vi "Preprocess_Data_for_TDMS.vi"(9 "Super Loop Index":i32, 10 "Previous Cluster":T2={"Meas Pressure"=[], "Meas Flowrate"=[], "Current Time"=0.0, "Start Time"=0.0, "Ref Pressure"=[], "Ref Flowrate"=[], "Flowrate Limits"={"Max"=300.0, "Min"=0.0}, "Chan 1 Gains"={"Kp"=0.0, "Ti"=0.0, "Td"=0.0}, "Chan 2 Gains"={"Kp"=0.0, "Ti"=0.0, "Td"=0.0}, "Chan 3 Gains"={"Kp"=0.0, "Ti"=0.0, "Td"=0.0}}, 11 "Current Cluster":T2={"Meas Pressure"=[], "Meas Flowrate"=[], "Current Time"=0.0, "Start Time"=0.0, "Ref Pressure"=[], "Ref Flowrate"=[], "Flowrate Limits"={"Max"=300.0, "Min"=0.0}, "Chan 1 Gains"={"Kp"=0.0, "Ti"=0.0, "Td"=0.0}, "Chan 2 Gains"={"Kp"=0.0, "Ti"=0.0, "Td"=0.0}, "Chan 3 Gains"={"Kp"=0.0, "Ti"=0.0, "Td"=0.0}}) -> (1 "appended array":bool[](array[boolean]), 2 "Contoler Change?":bool, 3 "output cluster":T1)   [LabVIEW 2021]
panel:
  out "initialized array":dbl[][](array[numeric])
  out "P":dbl[][](array[numeric])
  out "P array":dbl[][](array[numeric])
  out "Meas Pressure":dbl[](array[numeric])
  out "Ref Pressure":dbl[](array[numeric])
  out "FR":dbl[][](array[numeric])
  out "Ref P":dbl[][](array[numeric])
  out "Ref FR":dbl[][](array[numeric])
  out "Control":dbl[][](array[numeric])
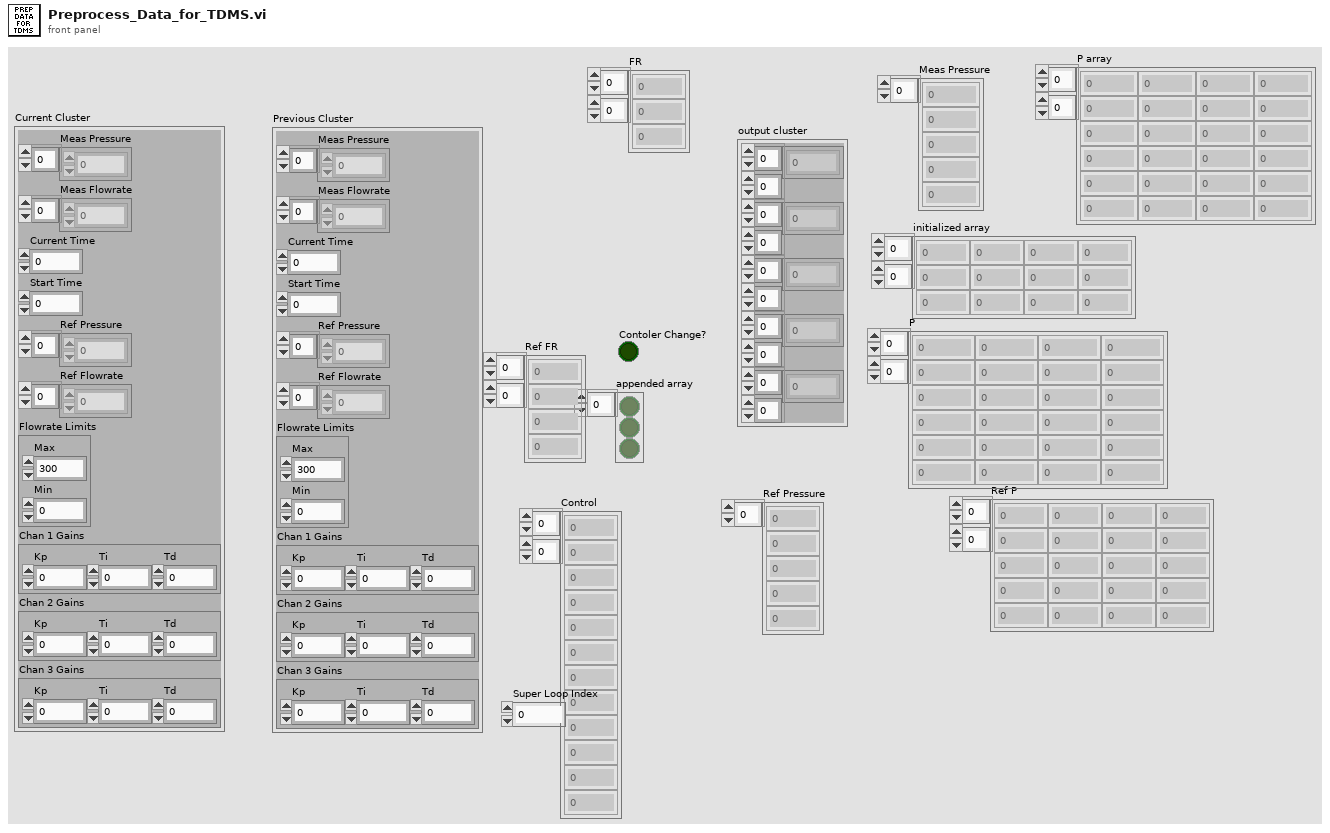
[diagram p1: front panel]
types:
  T1 = cluster{dbl[][], dbl[][], dbl[][], dbl[][], dbl[][]}
  T2 = cluster{"Meas Pressure":dbl[], "Meas Flowrate":dbl[], "Current Time":dbl, "Start Time":dbl, "Ref Pressure":dbl[], "Ref Flowrate":dbl[], "Flowrate Limits":cluster{"Max":dbl, "Min":dbl}, "Chan 1 Gains":cluster{"Kp":dbl, "Ti":dbl, "Td":dbl}, "Chan 2 Gains":cluster{"Kp":dbl, "Ti":dbl, "Td":dbl}, "Chan 3 Gains":cluster{"Kp":dbl, "Ti":dbl, "Td":dbl}}
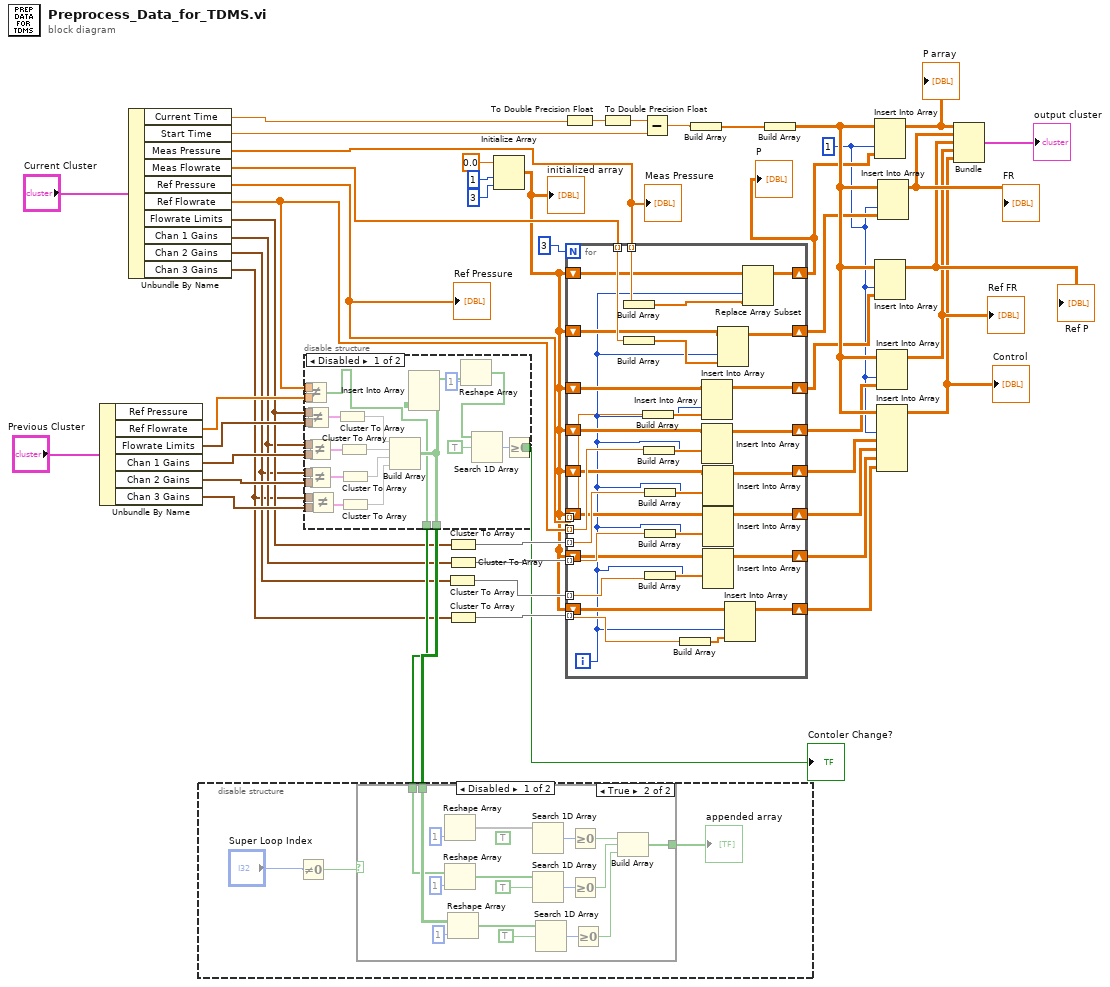
[diagram p0: block diagram]
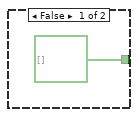
[diagram p3: hidden frame]
diagram:
  w1 = 1 ("disabled index (col)")
  n1 = Unbundle By Name("Previous Cluster") -> ("Ref Flowrate"=w37:dbl[], "Flowrate Limits"=w32:cluster{"Max":dbl, "Min":dbl}, "Chan 1 Gains"=w31:cluster{"Kp":dbl, "Ti":dbl, "Td":dbl}, "Chan 2 Gains"=w30:cluster{"Kp":dbl, "Ti":dbl, "Td":dbl}, "Chan 3 Gains"=w29:cluster{"Kp":dbl, "Ti":dbl, "Td":dbl})  [unwired: 1 out]
  n2 = Unbundle By Name("Current Cluster") -> ("Current Time"=w40:dbl, "Start Time"=w39:dbl, "Meas Pressure"=w13:dbl[], "Meas Flowrate"=w14:dbl[], "Ref Pressure"=w21:dbl[], "Ref Flowrate"=w10:dbl[], "Flowrate Limits"=w20:cluster{"Max":dbl, "Min":dbl}, "Chan 1 Gains"=w19:cluster{"Kp":dbl, "Ti":dbl, "Td":dbl}, "Chan 2 Gains"=w18:cluster{"Kp":dbl, "Ti":dbl, "Td":dbl}, "Chan 3 Gains"=w17:cluster{"Kp":dbl, "Ti":dbl, "Td":dbl})
  "Ref Pressure" <- w21
  "Meas Pressure" <- w13
  n3 = disable-structure shown="Disabled" {
    disable-tunnel: w37 -> [w75 _]
    disable-tunnel: w32 -> [w74 _]
    disable-tunnel: w31 -> [w73 _]
    disable-tunnel: w30 -> [w72 _]
    disable-tunnel: w29 -> [w71 _]
    disable-tunnel: [w70 _] -> w23
    disable-tunnel: [w69 _] -> w22
    disable-tunnel: w20 -> [w68 _]
    disable-tunnel: w19 -> [w67 _]
    disable-tunnel: w18 -> [w66 _]
    disable-tunnel: w17 -> [w65 _]
    disable-tunnel: [w64 _] -> w15
    disable-tunnel: w10 -> [w63 _]
    frame Disabled {
      n4 = Not Equal?(x=w63, y=w75) -> (x != y?=w69:bool[])
      n5 = Not Equal?(x=w68, y=w74) -> (x != y?=w62:cluster{"Max":bool, "Min":bool})
      n6 = Not Equal?(x=w67, y=w73) -> (x != y?=w61:cluster{"Kp":bool, "Ti":bool, "Td":bool})
      n7 = Not Equal?(x=w66, y=w72) -> (x != y?=w60:cluster{"Kp":bool, "Ti":bool, "Td":bool})
      n8 = Not Equal?(x=w65, y=w71) -> (x != y?=w59:cluster{"Kp":bool, "Ti":bool, "Td":bool})
      n9 = Cluster To Array(cluster=w62) -> (array=w53:bool[])
      n10 = Cluster To Array(cluster=w61) -> (array=w52:bool[])
      n11 = Cluster To Array(cluster=w60) -> (array=w51:bool[])
      n12 = Cluster To Array(cluster=w59) -> (array=w50:bool[])
      n13 = Build Array(w53, w52, w51, w50) -> (w70:bool[][])
      n14 = Insert Into Array(new element=w70) -> (w58:bool[])  [unwired: 3 in]
      n15 = Reshape Array(w58, 1 ("dimension size")) -> (w56:bool[])
      n16 = Search 1D Array(1D array=w56, element=TRUE) -> (index of element=w54:i32)  [unwired: 1 in]
      n17 = Greater Or Equal To 0?(x=w54) -> (x >= 0?=w64:bool)
    }
    frame Enabled {
    }
  }
  "Contoler Change?" <- w15
  n18 = disable-structure shown="Disabled" {
    disable-tunnel: w23 -> [w80 _]
    disable-tunnel: w22 -> [w79 _]
    frame Disabled {
      n19 = Not Equal To 0?(x="Super Loop Index") -> (x != 0?=w76:bool)
      n20 = case shown="True" w76 {
        tunnel: w80 -> [_ w84]
        tunnel: w79 -> [_ w83]
        tunnel: [bool[] [] w82] -> w78
        frame False {
        }
        frame True {
          (unwired) TRUE ("element")
          n21 = Reshape Array(1 ("dimension size")) -> (w96:void[])  [unwired: 1 in]
          n22 = Reshape Array(w83, 1 ("dimension size")) -> (w92:bool[])
          n23 = Reshape Array(w84, 1 ("dimension size")) -> (w88:bool[])
          n24 = Search 1D Array(1D array=w96) -> (index of element=w98:i32)  [unwired: 2 in]
          n25 = Search 1D Array(1D array=w92, element=TRUE) -> (index of element=w94:i32)  [unwired: 1 in]
          n26 = Search 1D Array(1D array=w88, element=TRUE) -> (index of element=w90:i32)  [unwired: 1 in]
          n27 = Greater Or Equal To 0?(x=w98) -> (x >= 0?=w85:bool)
          n28 = Greater Or Equal To 0?(x=w94) -> (x >= 0?=w86:bool)
          n29 = Greater Or Equal To 0?(x=w90) -> (x >= 0?=w87:bool)
          n30 = Build Array(w85, w86, w87) -> (w82:bool[])
        }
      }
      "appended array" <- w78
    }
    frame Enabled {
    }
  }
  n31 = Cluster To Array(cluster=w18) -> (array=w33:dbl[])
  n32 = Cluster To Array(cluster=w20) -> (array=w35:dbl[])
  n33 = Cluster To Array(cluster=w19) -> (array=w34:dbl[])
  n34 = Cluster To Array(cluster=w17) -> (array=w36:dbl[])
  n35 = Initialize Array(0.0 ("element"), 1 ("dimension size"), 3 ("dimension size")) -> (w9:dbl[][])
  "initialized array" <- w9
  n36 = To Double Precision Float(number=w40) -> (double precision float=w47:dbl)
  n37 = for {
    N: 3 -> [_]
    tunnel: w36 -> [w131] mode=indexing
    tunnel: w35 -> [w130] mode=indexing
    tunnel: w34 -> [w129] mode=indexing
    tunnel: w33 -> [w128] mode=indexing
    tunnel: w10 -> [w126] mode=indexing
    tunnel: w14 -> [w118] mode=indexing
    tunnel: w13 -> [w117] mode=indexing
    shift-right: [w102] -> w12
    shift-left: w9 -> [w101]
    shift-right: [w116] -> w8
    shift-left: w9 -> [w115]
    tunnel: w21 -> [w127] mode=indexing
    shift-right: [w105] -> w7
    shift-left: w9 -> [w114]
    shift-right: [w112] -> w6
    shift-left: w9 -> [w113]
    shift-right: [w110] -> w5
    shift-left: w9 -> [w111]
    shift-right: [w108] -> w4
    shift-left: w9 -> [w109]
    shift-right: [w106] -> w3
    shift-left: w9 -> [w107]
    shift-right: [w103] -> w2
    shift-left: w9 -> [w104]
    i -> [w99]
    n38 = Build Array(w117) -> (w100:dbl[])
    n39 = Build Array(w118) -> (w119:dbl[])
    n40 = Build Array(w127) -> (w125:dbl[])
    n41 = Build Array(w126) -> (w124:dbl[])
    n42 = Build Array(w130) -> (w123:dbl[])
    n43 = Build Array(w129) -> (w122:dbl[])
    n44 = Build Array(w128) -> (w121:dbl[])
    n45 = Build Array(w131) -> (w120:dbl[])
    n46 = Insert Into Array(array=w114, index (col)=w99, new element=w125) -> (w105:dbl[][])  [unwired: 1 in]
    n47 = Insert Into Array(array=w113, index (col)=w99, new element=w124) -> (w112:dbl[][])  [unwired: 1 in]
    n48 = Insert Into Array(array=w111, index (col)=w99, new element=w123) -> (w110:dbl[][])  [unwired: 1 in]
    n49 = Insert Into Array(array=w109, index (col)=w99, new element=w122) -> (w108:dbl[][])  [unwired: 1 in]
    n50 = Insert Into Array(array=w107, index (col)=w99, new element=w121) -> (w106:dbl[][])  [unwired: 1 in]
    n51 = Insert Into Array(array=w115, index (col)=w99, new element=w119) -> (w116:dbl[][])  [unwired: 1 in]
    n52 = Insert Into Array(array=w104, index (col)=w99, new element=w120) -> (w103:dbl[][])  [unwired: 1 in]
    n53 = Replace Array Subset(array=w101, new element=w100, index (col)=w99) -> (w102:dbl[][])  [unwired: 1 in]
  }
  "P" <- w12
  n54 = To Double Precision Float(number=w47) -> (double precision float=w46:dbl)
  n55 = Subtract(x=w46, y=w39) -> (x-y=w48:dbl)
  n56 = Build Array(w48) -> (w49:dbl[])
  n57 = Build Array(w49) -> (w28:dbl[][])
  n58 = Insert Into Array(array=w28, index (col)=w1, new element=w12) -> (w43:dbl[][])  [unwired: 1 in]
  "P array" <- w43
  n59 = Insert Into Array(array=w28, index (col)=w1, new element=w7) -> (w27:dbl[][])  [unwired: 1 in]
  "Ref P" <- w27
  n60 = Insert Into Array(array=w28, index (col)=w1, new element=w6) -> (w26:dbl[][])  [unwired: 1 in]
  "Ref FR" <- w26
  n61 = Insert Into Array(array=w28, index (col)=w1, new element #1=w5, new element #2=w4, new element #3=w3, new element #4=w2) -> (w25:dbl[][])  [unwired: 1 in]
  "Control" <- w25
  n62 = Insert Into Array(array=w28, index (col)=w1, new element=w8) -> (w42:dbl[][])  [unwired: 1 in]
  "FR" <- w42
  n63 = Bundle(w43, w42, w27, w26, w25) -> (→"output cluster":T1)  [unwired: 1 in]
